vi "Create Chans.vi"(5 "New Section Name (none)":string, 6 "new section GUID (\"\":del prot)":string, 7 "Type":T3=enum."Output", 8 "error in (no error)":errorcluster, 10 "Channels":T2[](array[typedef]), 11 "Section Ptr":T1 format="%.0x") -> (0 "error out":errorcluster, 1 "new channel references":T1[](array[typedef]) format="%.0x", 2 "new section ref":T1=18446744073709551615 format="%.0x", 3 "Section Ptr dup":T1 format="%.0x")   [LabVIEW 2015, in "Engine Simulation Toolkit System Explorer.lvlib"]
uses:
  Engine Simulation Toolkit System Explorer.lvlib
  <vilib>/NI Veristand/Custom Device API/Custom Device Item Ref.ctl
  <vilib>/NI Veristand/Custom Device API/Custom Device Channel Type.ctl
  Shared/Channel.ctl
  <vilib>/NI Veristand/Custom Device API/Custom Device Channel.ctl
  Shared/Constants and GUIDs.vi
  <vilib>/NI Veristand/Custom Device API/Custom Device API.lvlib
  Shared/Engine Simulation Toolkit Shared.lvlib
  <vilib>/NI/NI VeriStand Advanced SysDef API/SysDef API/Advanced System Definition.lvlib
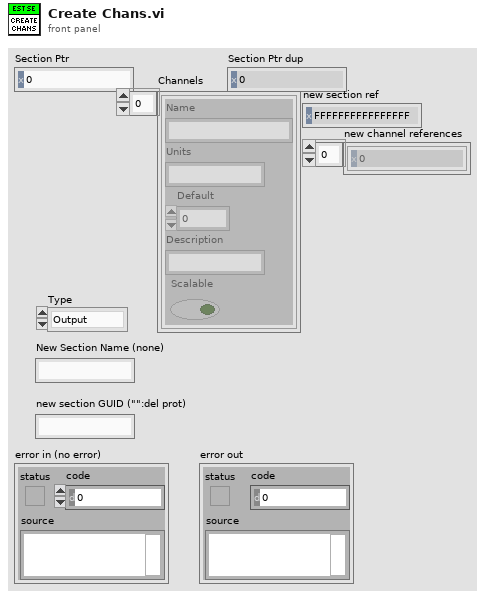
[diagram p1: front panel]
types:
  T1 = typedef "Custom Device API.lvlib/Custom Device Item Ref.ctl" = u64
  T2 = typedef "Engine Simulation Toolkit Shared.lvlib/Channel.ctl" = cluster{"Name":string, "Units":string, "Default":dbl, "Description":string, "Scalable":bool}
  T3 = typedef "Custom Device API.lvlib/Custom Device Channel Type.ctl" = enum16{"Input", "Output"}
  T4 = typedef "Custom Device API.lvlib/Custom Device Channel.ctl" = cluster{"Type":T3, "Units":string, "Default Value":dbl, "Faultable":bool, "Scalable":bool}
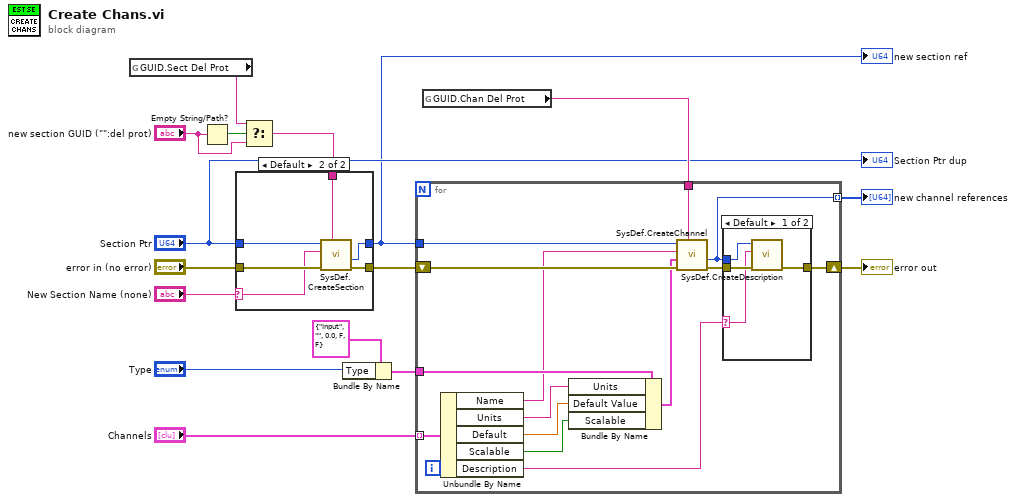
[diagram p0: block diagram]
diagram:
  n1 = global read "Constants and GUIDs.vi" "GUID.Sect Del Prot"() -> (w4:string)
  n2 = Empty String/Path?(string/path="new section GUID (\"\":del prot)") -> (empty?=w5:bool)
  n3 = Select(t=w4, s=w5, f="new section GUID (\"\":del prot)") -> (s? t:f=w2:string)
  n4 = case shown="Default" "New Section Name (none)" {
    selector: "New Section Name (none)" -> [_ w20]
    tunnel: "error in (no error)" -> [w18 w24]
    tunnel: "Section Ptr" -> [w17 w23]
    tunnel: [w18 w22] -> w9
    tunnel: [w17 w21] -> w8
    tunnel: w2 -> [_ w19]
    frame "" {
    }
    frame Default {
      n5 = call <vilib>:"SysDef.CreateSection.vi"("GUID"=w19, "error in (no error)"=w24, "Name"=w20, "nodeID"=w23) -> ("error out"=w22:errorcluster, "New NodeID"=w21:u64)  [unwired: 4 in, 2 out]
    }
  }
  "new section ref" <- w8
  n6 = Bundle By Name(cluster=T4 {"Type"=enum."Input", "Units"="", "Default Value"=0.0, "Faultable"=FALSE, "Scalable"=FALSE} ("Channel"), "Type"="Type") -> (w10:T4)
  n7 = global read "Constants and GUIDs.vi" "GUID.Chan Del Prot"() -> (w16:string)
  n8 = for {
    tunnel: w8 -> [w37]
    shift-right: [w33] -> w14
    shift-left: w9 -> [w38]
    tunnel: w10 -> [w36]
    tunnel: w16 -> [w34]
    tunnel: "Channels" -> [w31] mode=indexing
    tunnel: [w26] -> w1 mode=indexing
    n9 = Unbundle By Name(w31) -> ("Name"=w30:string, "Units"=w29:string, "Default"=w28:dbl, "Scalable"=w25:bool, "Description"=w27:string)
    n10 = Bundle By Name(cluster=w36, "Units"=w29, "Default Value"=w28, "Scalable"=w25) -> (w35:T4)
    n11 = call <vilib>:"SysDef.CreateChannel.vi"("GUID"=w34, "error in (no error)"=w38, "Channel"=w35, "Name"=w30, "nodeID"=w37) -> ("error out"=w32:errorcluster, "New NodeID"=w26:u64)  [unwired: 3 in, 2 out]
    n12 = case shown="Default" w27 {
      selector: w27 -> [w39 _]
      tunnel: [w41 w43] -> w33
      tunnel: w32 -> [w42 w43]
      tunnel: w26 -> [w40 _]
      frame Default {
        n13 = call <vilib>:"SysDef.CreateDescription.vi"("error in (no error)"=w42, "Description"=w39, "ID in"=w40) -> ("error out"=w41:errorcluster)  [unwired: 7 in, 1 out]
      }
      frame "" {
      }
    }
  }
  "error out" <- w14
  "new channel references" <- w1
  "Section Ptr dup" <- "Section Ptr"
